vi "Text File Data Finder.vi"(11 "File Path Control":path) -> (1 "Total Amount of Points":dbl, 2 "Sample Rate":dbl, 3 "File Path Indicator":path)   [LabVIEW 2014]
panel:
  # "Text File Finder"
  # "Inputs"
  # "Output"
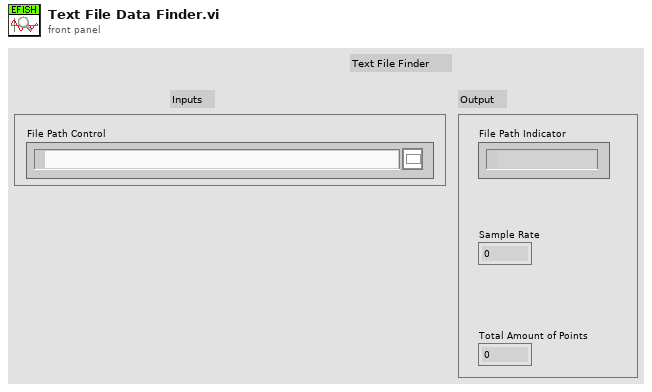
[diagram p1: front panel]
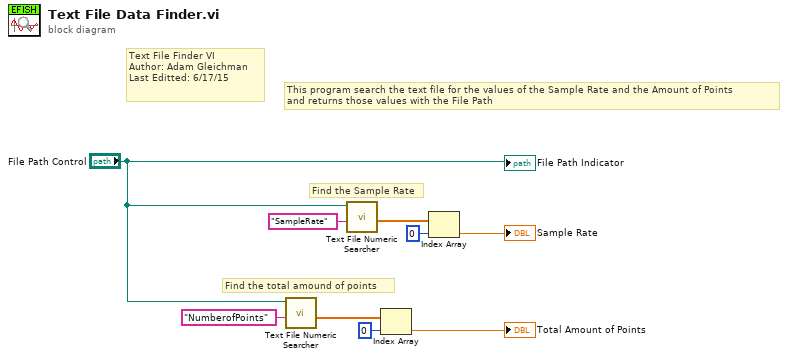
[diagram p0: block diagram]
diagram:
  # "This program search the text file for the values of the Sample Rate and the Amount of Points\nand returns those values with the File Path"
  # "Text File Finder VI\nAuthor: Adam Gleichman\nLast Editted: 6/17/15"
  # "Find the total amound of points"
  # "Find the Sample Rate"
  n1 = call "Text File Numeric Searcher.vi"("String"="NumberofPoints", "file (use dialog)"="File Path Control") -> ("Numeric Array"=w6:dbl[])  [unwired: 8 in, 1 out]
  n2 = call "Text File Numeric Searcher.vi"("String"="SampleRate", "file (use dialog)"="File Path Control") -> ("Numeric Array"=w3:dbl[])  [unwired: 8 in, 1 out]
  n3 = Index Array(array=w6, index=0) -> (element=→"Total Amount of Points":dbl)
  n4 = Index Array(array=w3, index=0) -> (element=→"Sample Rate":dbl)
  "File Path Indicator" <- "File Path Control"
